vi "Filter Event Data.vi"(8 "error in (no error)":errorcluster, 10 "EventFilter Reference":T1, 11 "MenuActivationMsg in":refnum<class "MenuActivationMsg.lvclass">) -> (0 "error out":errorcluster, 2 "Discard?":bool, 3 "MenuActivationMsg out":refnum<class "MenuActivationMsg.lvclass">)   [LabVIEW 2020, in "ActorEvents.lvlib" / "MenuActivationMsg.lvclass"]
uses:
  <vilib>/gpm_packages/@cs/mva-viewable/Source/ActorEvents/IEventAggregator Messages/Menu Activation Msg/MenuActivationMsg.lvclass
  <vilib>/gpm_packages/@cs/mva-viewable/Source/ActorEvents/IEventFilter/EventFilter Reference.ctl
  <vilib>/gpm_packages/@cs/mva-viewable/Source/ActorEvents/IEventFilter/IEventFilter.lvclass
  <vilib>/gpm_packages/@cs/mva-viewable/Source/ActorEvents/IEventAggregator Messages/Menu Activation Msg/MenuActivationMsg.lvclass/MenuActivationMsg.ctl
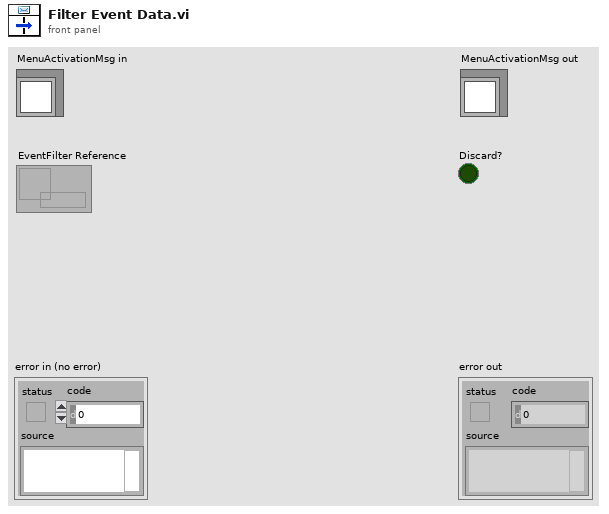
[diagram p1: front panel]
types:
  T1 = typedef "ActorEvents.lvlib/IEventFilter.lvclass/EventFilter Reference.ctl" = refnum<data-value>
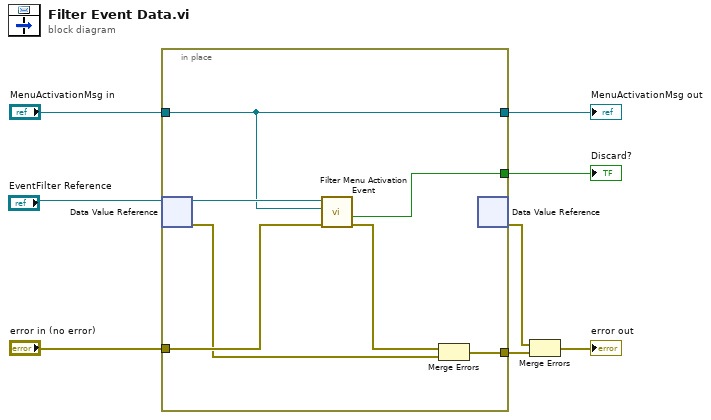
[diagram p0: block diagram]
diagram:
  n1 = in-place {
    in-place-border: "MenuActivationMsg in" -> [w9]
    in-place-border: "error in (no error)" -> [w14]
    in-place-border: [w13] -> w5
    in-place-border: [w11] -> w4
    in-place-border: [w9] -> w3
    n2 = in-place-dvr #1("EventFilter Reference") -> (w15:refnum<class "IEventFilter.lvclass">, w10:errorcluster)
    n3 = call-dynamic "Filter Menu Activation Event.vi"("error in (no error)"=w14, "MenuActivationMsg"=w9, "IEventFilter in"=w15) -> ("error out"=w12:errorcluster, "Discard?"=w13:bool)  [unwired: 6 in, 1 out]
    n4 = Merge Errors(w12, w10) -> (w11:errorcluster)
    n5 = in-place-dvr #1() -> (w1:errorcluster)  [unwired: 1 in, 1 out]
  }
  "MenuActivationMsg out" <- w3
  "Discard?" <- w5
  n6 = Merge Errors(w1, w4) -> (→"error out":errorcluster)
